vi "Vision.vi"() -> (0 "error out":errorcluster)   [LabVIEW 2016]
uses:
  <vilib>/vision/NI_Vision_Development_Module.lvlib
panel:
  out "Image 2":T1(plugin-control)
  out "Original Image":T1(plugin-control)
  out "Image":T1(plugin-control)
  out "프레임 rate":dbl
  in  "이미지 형식":T2 items=["Grayscale (U8)", "Grayscale (I16)", "Grayscale (SGL)", "Complex (CSG)", "RGB (U32)", "HSL (U32)", "RGB (U64)", "Grayscale (U16)"]
  in  "Stop?":bool
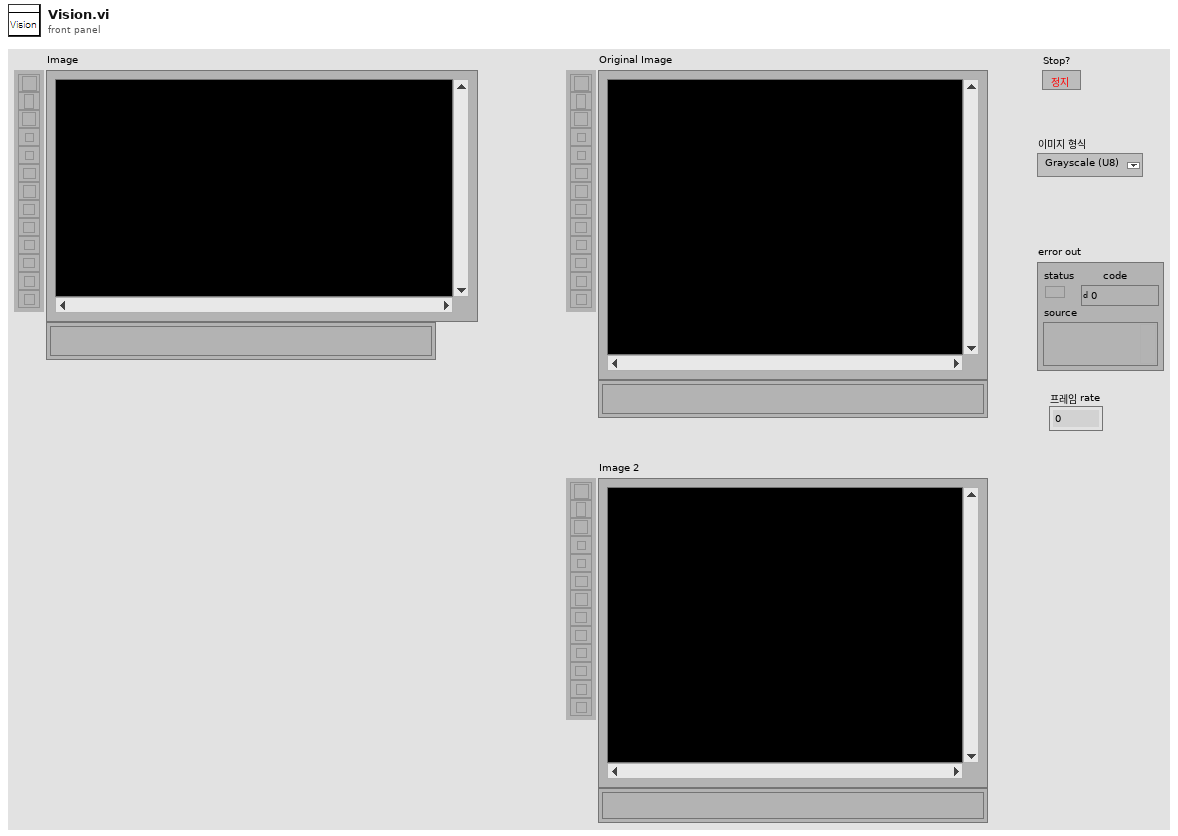
[diagram p1: front panel]
types:
  T1 = typedef "IMAQ Image.ctl" = refnum<image>
  T2 = typedef "Image Type" = u32
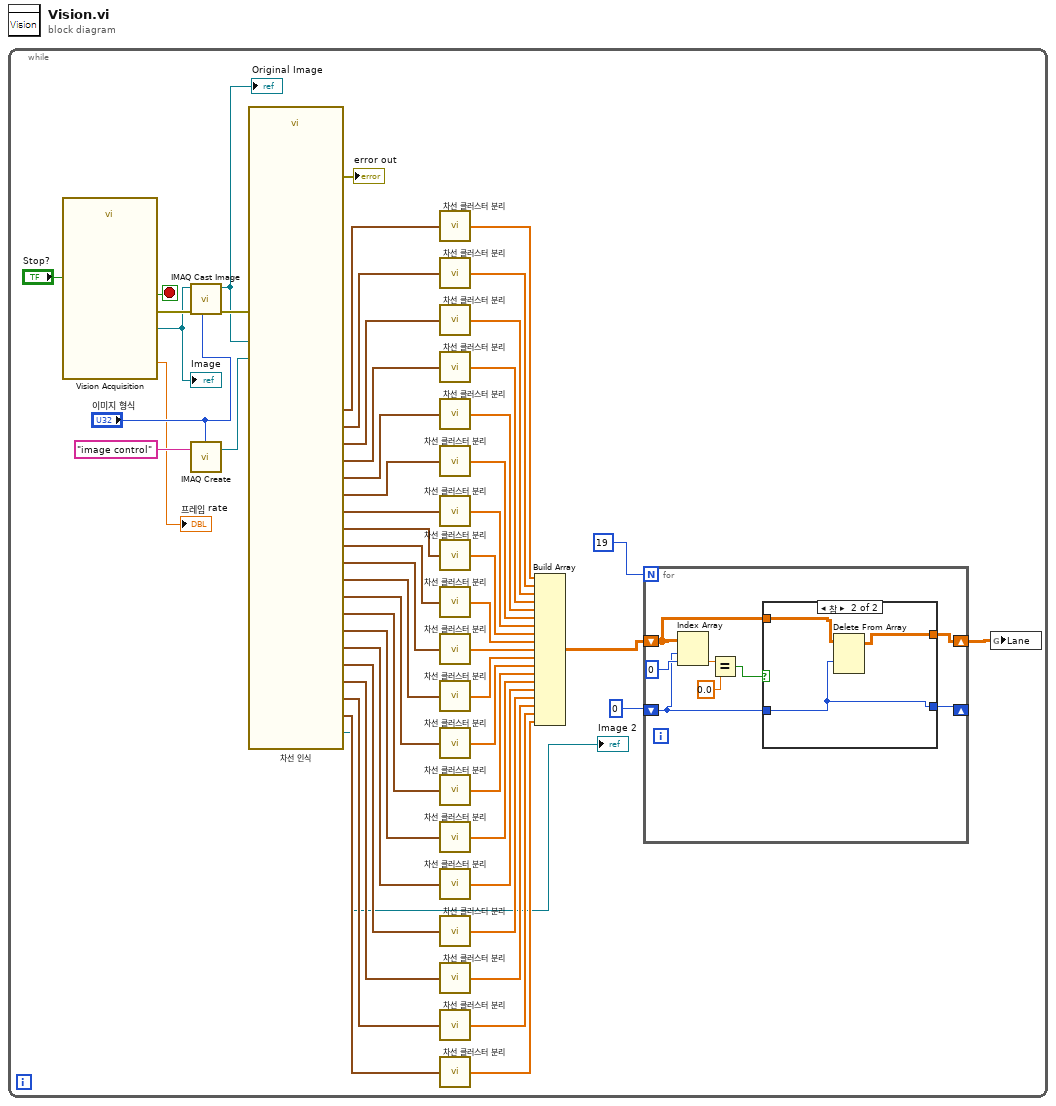
[diagram p0: block diagram]
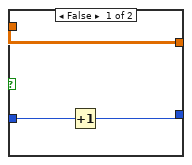
[diagram p2: hidden frame]
diagram:
  n1 = while {
    stop <- w6 stop-if-true
    n2 = call "Vision Acquisition"("Stop (F)"="Stop?") -> ("Image Out"=w45:T1, "Frame Rate"=→"프레임 rate":dbl, "Stopped"=w6:bool, "error out"=w51:errorcluster)  [unwired: 23 in]
    "Image" <- w45
    n3 = call "IMAQ Cast Image"("Image Type"="이미지 형식", "error in (no error)"=w51, "Image Src"=w45) -> ("error out"=w50:errorcluster, "Image Dst Out"=w46:T1)  [unwired: 7 in]
    "Original Image" <- w46
    n4 = call "IMAQ Create"("Image Name"="image control", "Image Type"="이미지 형식") -> ("New Image"=w47:T1)  [unwired: 3 in, 1 out]
    n5 = call "차선 인식"("Image In"=w46, "Image Dst"=w47, "error in"=w50) -> ("Edges Coordinates (calibrated) (Edge Detector 21)"=w24:cluster{"X":sgl, "Y":sgl}[], "Edges Coordinates (calibrated) (Edge Detector 20)"=w25:cluster{"X":sgl, "Y":sgl}[], "Edges Coordinates (calibrated) (Edge Detector 19)"=w26:cluster{"X":sgl, "Y":sgl}[], "Edges Coordinates (calibrated) (Edge Detector 18)"=w27:cluster{"X":sgl, "Y":sgl}[], "Edges Coordinates (calibrated) (Edge Detector 14)"=w28:cluster{"X":sgl, "Y":sgl}[], "Edges Coordinates (calibrated) (Edge Detector 17)"=w29:cluster{"X":sgl, "Y":sgl}[], "Edges Coordinates (calibrated) (Edge Detector 16)"=w30:cluster{"X":sgl, "Y":sgl}[], "Edges Coordinates (calibrated) (Edge Detector 15)"=w31:cluster{"X":sgl, "Y":sgl}[], "Edges Coordinates (calibrated) (Edge Detector 13)"=w32:cluster{"X":sgl, "Y":sgl}[], "Edges Coordinates (calibrated) (Edge Detector 12)"=w33:cluster{"X":sgl, "Y":sgl}[], "Edges Coordinates (calibrated) (Edge Detector 11)"=w34:cluster{"X":sgl, "Y":sgl}[], "Edges Coordinates (calibrated) (Edge Detector 10)"=w35:cluster{"X":sgl, "Y":sgl}[], "Edges Coordinates (calibrated) (Edge Detector 8)"=w36:cluster{"X":sgl, "Y":sgl}[], "Edges Coordinates (calibrated) (Edge Detector 7)"=w37:cluster{"X":sgl, "Y":sgl}[], "Edges Coordinates (calibrated) (Edge Detector 5)"=w38:cluster{"X":sgl, "Y":sgl}[], "Image Out"=→"Image 2":T1, "Edges Coordinates (calibrated) (Edge Detector 1)"=w44:cluster{"X":sgl, "Y":sgl}[], "Edges Coordinates (calibrated) (Edge Detector 2)"=w42:cluster{"X":sgl, "Y":sgl}[], "Edges Coordinates (calibrated) (Edge Detector 3)"=w40:cluster{"X":sgl, "Y":sgl}[], "Edges Coordinates (calibrated) (Edge Detector 4)"=w39:cluster{"X":sgl, "Y":sgl}[], "error out"=→"error out":errorcluster)  [unwired: 2 in, 2 out]
    n6 = call "차선 클러스터 분리.vi"("배열"=w44) -> ("R, Theta"=w43:dbl[])
    n7 = call "차선 클러스터 분리.vi"("배열"=w42) -> ("R, Theta"=w41:dbl[])
    n8 = call "차선 클러스터 분리.vi"("배열"=w40) -> ("R, Theta"=w23:dbl[])
    n9 = call "차선 클러스터 분리.vi"("배열"=w39) -> ("R, Theta"=w22:dbl[])
    n10 = call "차선 클러스터 분리.vi"("배열"=w38) -> ("R, Theta"=w21:dbl[])
    n11 = call "차선 클러스터 분리.vi"("배열"=w37) -> ("R, Theta"=w20:dbl[])
    n12 = call "차선 클러스터 분리.vi"("배열"=w36) -> ("R, Theta"=w19:dbl[])
    n13 = call "차선 클러스터 분리.vi"("배열"=w35) -> ("R, Theta"=w18:dbl[])
    n14 = call "차선 클러스터 분리.vi"("배열"=w34) -> ("R, Theta"=w17:dbl[])
    n15 = call "차선 클러스터 분리.vi"("배열"=w33) -> ("R, Theta"=w16:dbl[])
    n16 = call "차선 클러스터 분리.vi"("배열"=w32) -> ("R, Theta"=w15:dbl[])
    n17 = call "차선 클러스터 분리.vi"("배열"=w31) -> ("R, Theta"=w14:dbl[])
    n18 = call "차선 클러스터 분리.vi"("배열"=w30) -> ("R, Theta"=w13:dbl[])
    n19 = call "차선 클러스터 분리.vi"("배열"=w29) -> ("R, Theta"=w12:dbl[])
    n20 = call "차선 클러스터 분리.vi"("배열"=w28) -> ("R, Theta"=w11:dbl[])
    n21 = call "차선 클러스터 분리.vi"("배열"=w27) -> ("R, Theta"=w10:dbl[])
    n22 = call "차선 클러스터 분리.vi"("배열"=w26) -> ("R, Theta"=w9:dbl[])
    n23 = call "차선 클러스터 분리.vi"("배열"=w25) -> ("R, Theta"=w8:dbl[])
    n24 = call "차선 클러스터 분리.vi"("배열"=w24) -> ("R, Theta"=w7:dbl[])
    n25 = Build Array(w43, w41, w23, w22, w21, w20, w19, w18, w17, w16, w15, w14, w13, w12, w11, w10, w9, w8, w7) -> (w3:dbl[][])
    n26 = for {
      N: 19 -> [_]
      shift-right: [w57] -> _
      shift-left: 0 -> [w55]
      shift-right: [w56] -> w2
      shift-left: w3 -> [w58]
      n27 = Index Array(array=w58, index (row)=w55, index (col)=0 ("비활성화된 인덱스 (열)")) -> (element=w61:dbl)
      n28 = Equal?(x=w61, y=0.0) -> (x = y?=w59:bool)
      n29 = case shown="참" w59 {
        tunnel: w58 -> [w65 w68]
        tunnel: [w65 w66] -> w56
        tunnel: w55 -> [w64 w67]
        tunnel: [w63 w67] -> w57
        frame False {
          n30 = Increment(x=w64) -> (x+1=w63:i32)
        }
        frame True {
          n31 = Delete From Array(array=w68, index (row)=w67) -> (array with subset deleted=w66:dbl[][])  [unwired: 2 in, 1 out]
        }
      }
    }
    n32 = global write "[GV]_Vision Lane.vi" "Lane"(w2) -> ()
  }
